vi "MeasurePower.vi"(0 "object in":refnum<class "AD2_SDK.lvclass">, 3 "Voltage Probe Scaling(V/A)":dbl, 5 "error in (no error)":errorcluster) -> (14 "object out":refnum<class "AD2_SDK.lvclass">, 15 "Power (W)":dbl format="%0.2p", 16 "Impedance":dbl, 17 "Phase (deg)":dbl, 18 "Channels array":waveform(dbl)[](array[waveform]), 19 "error out":errorcluster)   [LabVIEW 2023, in "AD2_SDK.lvclass"]
uses:
  AD2_SDK.lvclass
  <vilib>/measure/matone.llb/Extract Single Tone Information 1 Chan.vi
  <vilib>/measure/madcrms.llb/Basic Averaged DC-RMS for 1 Chan.vi
  AD2_SDK.lvclass/AD2_SDK.ctl
  <vilib>/measure/NI_MAPro.lvlib
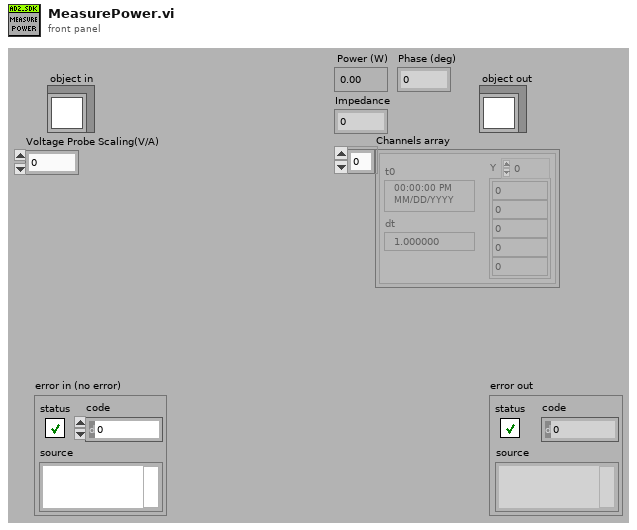
[diagram p1: front panel]
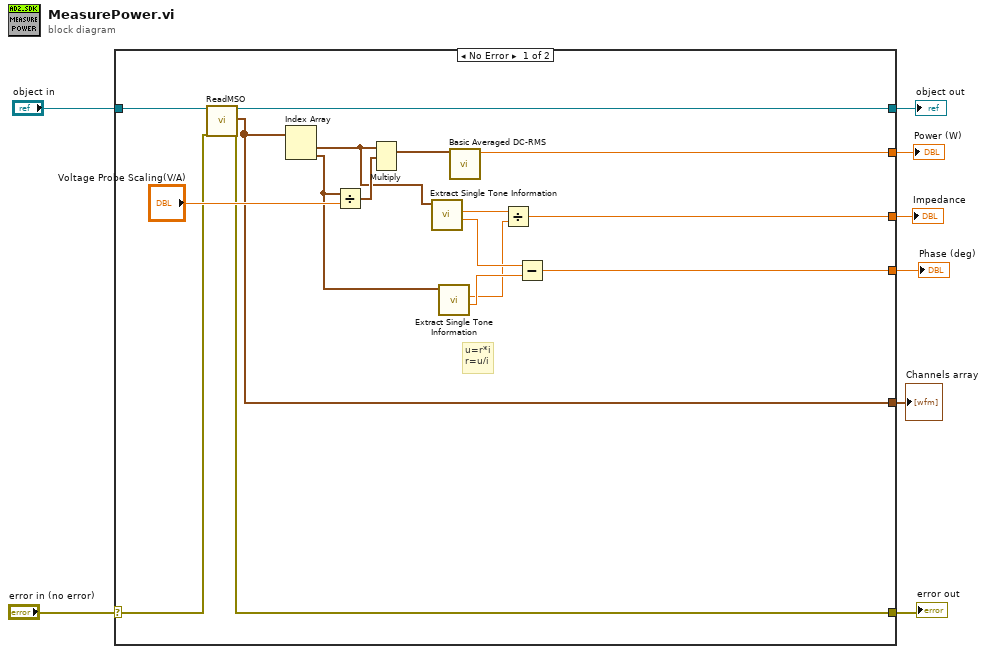
[diagram p0: block diagram]
diagram:
  n1 = case shown="No Error" "error in (no error)" {
    selector: "error in (no error)" -> [w11 w27]
    tunnel: [w10 w27] -> w7
    tunnel: [w25 w26] -> w5
    tunnel: "object in" -> [w24 w26]
    tunnel: [w14 _] -> w4
    tunnel: [w13 _] -> w3
    tunnel: [w12 _] -> w2
    tunnel: [w9 _] -> w1
    frame No Error {
      # "u=r*i\nr=u/i"
      n2 = call-dynamic "ReadMSO.vi"("object in"=w24, "error in (no error)"=w11) -> ("object out"=w25:refnum<class "AD2_SDK.lvclass">, "Channels array"=w9:waveform(dbl)[], "error out"=w10:errorcluster)  [unwired: 15 in]
      n3 = Index Array(array=w9) -> (element #1=w20:waveform(dbl), element #2=w19:waveform(dbl))  [unwired: 2 in]
      n4 = Divide(x=w19, y="Voltage Probe Scaling(V/A)") -> (x/y=w23:waveform(dbl))
      n5 = Multiply(1:w23, 2:w20) -> (0:w21:waveform(dbl))  [unwired: 1 in, 1 out]
      n6 = call-poly <vilib>:"Extract Single Tone Information.vi"("time signal in"=w20) -> ("detected phase (deg)"=w18:dbl, "detected amplitude"=w16:dbl)  [unwired: 5 in, 4 out]
      n7 = call-poly <vilib>:"Extract Single Tone Information.vi"("time signal in"=w19) -> ("detected phase (deg)"=w17:dbl, "detected amplitude"=w15:dbl)  [unwired: 5 in, 4 out]
      n8 = call-poly <vilib>:"Basic Averaged DC-RMS.vi"("signal in"=w21) -> ("DC value"=w12:dbl)  [unwired: 7 in, 3 out]
      n9 = Divide(x=w16, y=w15) -> (x/y=w13:dbl)
      n10 = Subtract(x=w18, y=w17) -> (x-y=w14:dbl)
    }
    frame Error {
    }
  }
  "error out" <- w7
  "object out" <- w5
  "Power (W)" <- w2
  "Impedance" <- w3
  "Phase (deg)" <- w4
  "Channels array" <- w1
